vi "PH_Powermeter_BaseClass.set current Setting to GUI.vi"(0 "VI in":refnum<vi>, 5 "error in (no error)":errorcluster) -> (14 "VI out":refnum<vi>, 19 "error out":errorcluster)   [LabVIEW 2014, in "PH_Powermeter_BaseClass.lvlib"]
uses:
  PH_Powermeter_BaseClass.lvlib
  PH_Common/PH_Common.lvlib
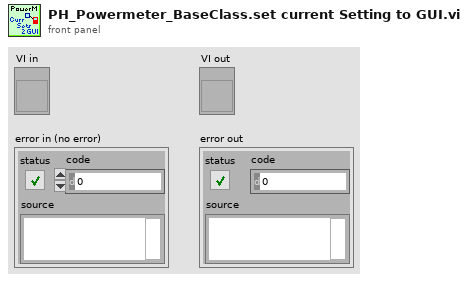
[diagram p1: front panel]
types:
  T1 = typedef "PH_Powermeter_BaseClass.lvlib/PH_Powermeter_BaseClass.i attribute.ctl" = cluster{"GUI References":T2, "Connection":T3, "Head Attributes":T5, "VISA resource":refnum<visa-resource-name>, "Energy":T6, "Service ID Energy":i32, "Wanted Settings":T7, "Current Settings":T7}
  T2 = typedef "PH_Powermeter_BaseClass.lvlib/PH_Powermeter_BaseClass.GUI Refs.ctl" = cluster{"Head Attributes":refnum<vi>, "Energy":refnum<vi>, "Connection":refnum<vi>, "VISA Resource":refnum<vi>, "Scaling Factor":refnum<vi>, "Range":refnum<vi>, "Wavelength":refnum<vi>, "Trigger Level":refnum<vi>, "Wanted Settings":refnum<vi>, "Current Settings":refnum<vi>}
  T3 = typedef "PH_Powermeter_BaseClass.lvlib/PH_Powermeter_BaseClass.Connection.ctl" = cluster{"failed checks":i8, "Timeout":bool, "Data read":string, "Failure":bool, "Error":bool, "State":T4}
  T4 = typedef "PH_Powermeter_BaseClass.lvlib/PH_Powermeter_BaseClass.State.ctl" = enum32{"off", "operating", "opened", "checked", "connected", "Sets to change", "running"}
  T5 = typedef "PH_Powermeter_BaseClass.lvlib/PH_Powermeter_BaseClass.Head Attributes.ctl" = cluster{"Instrument Type":string, "Head Version":string, "Head Name":string, "Serial Number":string, "Firmware":string, "Sensor Type":string, "MinimumRange":u32, "Maximum Range":u32, "Min Wavelength":i32, "Max Wavelength":i32}
  T6 = typedef "PH_Powermeter_BaseClass.lvlib/PH_Powermeter_BaseClass.Energy.ctl" = cluster{"current Value":dbl, "unscaled":dbl, "Scaling Factor":dbl}
  T7 = typedef "PH_Powermeter_BaseClass.lvlib/PH_gentec_BaseClass.Head Settings.ctl" = cluster{"Trigger Level":dbl, "Wavelength":u32, "Range":u32}
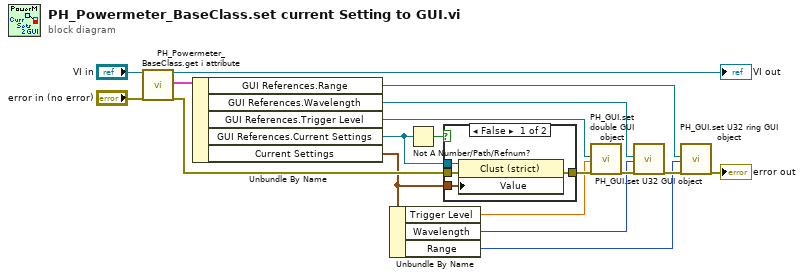
[diagram p0: block diagram]
diagram:
  n1 = call "PH_Powermeter_BaseClass.get i attribute.vi"("i ref in"="VI in", "error in (no error)"="error in (no error)") -> ("i ref out"=→"VI out":refnum<vi>, "i attribute"=w13:T1, "error out"=w18:errorcluster)  [unwired: 15 in]
  n2 = Unbundle By Name(w13) -> ("GUI References.Range"=w3:refnum<vi>, "GUI References.Wavelength"=w2:refnum<vi>, "GUI References.Trigger Level"=w1:refnum<vi>, "GUI References.Current Settings"=w11:refnum<vi>, "Current Settings"=w10:T7)
  n3 = Unbundle By Name(w10) -> ("Trigger Level"=w6:dbl, "Wavelength"=w5:u32, "Range"=w4:u32)
  n4 = Not A Number/Path/Refnum?(number/path/refnum=w11) -> (NaN/Path/Refnum?=w12:bool)
  n5 = case shown="False" w12 {
    tunnel: w18 -> [w22 w23]
    tunnel: [w21 w23] -> w14
    tunnel: w11 -> [w20 _]
    tunnel: w10 -> [w19 _]
    frame False {
      n6 = property class="Clust (strict)"(reference=w20, error in=w22, "Value"=w19) -> (error out=w21:errorcluster)  [unwired: 1 out]
    }
    frame True {
    }
  }
  n7 = call "PH_GUI.set double GUI object.vi"("GUI object Ref"=w1, "value"=w6, "error in (no error)"=w14) -> ("error out"=w9:errorcluster)  [unwired: 16 in]
  n8 = call "PH_GUI.set U32 GUI object.vi"("U32 Ref"=w2, "Value"=w5, "error in (no error)"=w9) -> ("error out"=w8:errorcluster)  [unwired: 16 in]
  n9 = call "PH_GUI.set U32 ring GUI object.vi"("Ring Ref"=w3, "Value"=w4, "error in (no error)"=w8) -> ("error out"=→"error out":errorcluster)  [unwired: 16 in]
